vi "Init sm Measurement.vi"(4 "Enable Buffering (Enable)":bool, 5 "Sample Rate (1000 Hz)":i32=1000, 6 "Number of Acquisitions (100)":i32=100, 7 "Trigger Type (0:Untriggered)":u16(ring)=2 items=["Untriggered", "Software Triggered", "Hardware Triggered"], 8 "error in (no error)":errorcluster, 9 "Trigger Stop Condition (1:Edge Triggering)":u16(ring)=1 items=["Number of Acquisitions", "Edge Triggering"], 10 "Enable Unbuffered Data (Enabled)":bool=TRUE, 11 "Micron sm Digitizer in":refnum<class "Micron sm Digitizer.lvclass">) -> (0 "error out":errorcluster, 2 "Number of Sensors":u16[](array[numeric]), 3 "Micron sm Digitizer out":refnum<class "Micron sm Digitizer.lvclass">)   [LabVIEW 2024, in "Micron sm Digitizer.lvclass"]
uses:
  Micron sm Digitizer.lvclass
  D:/GitHub/NHMFL_Core/Libraries/Instruments/VISA Instrument/VISA Instrument.lvclass
  D:/GitHub/NHMFL_Core/Libraries/Instruments/Micron Optics/Micron Optics Driver/Micron Optics Driver.lvclass
  VISA Instrument/VISA Instrument.lvclass/VISA Instrument.ctl
  VISA Instrument/Read VISA resource.vi
  VISA Instrument/Write VISA resource.vi
  Micron sm Digitizer.lvclass/Micron sm Digitizer.ctl
  Micron Optics sm130/Micron Optics sm130.lvlib
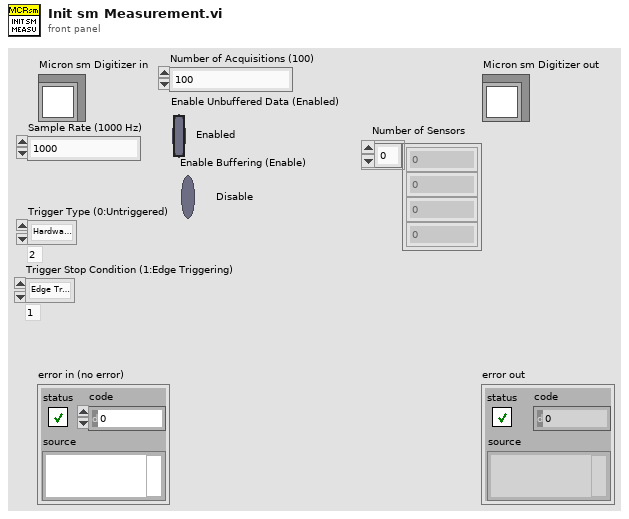
[diagram p1: front panel]
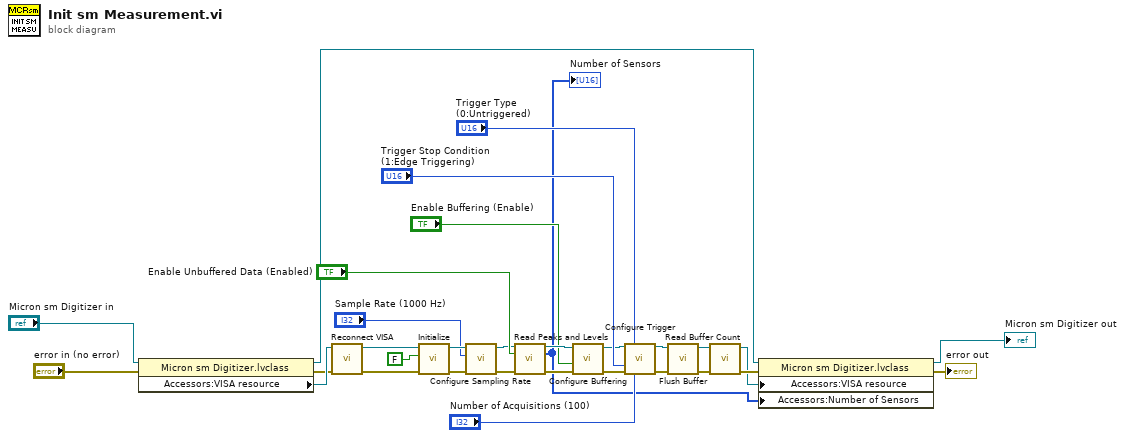
[diagram p0: block diagram]
diagram:
  n1 = property class="Micron sm Digitizer.lvclass"(reference="Micron sm Digitizer in", error in="error in (no error)") -> (reference out=w26:refnum<class "Micron sm Digitizer.lvclass">, error out=w2:errorcluster, "Accessors:VISA resource"=w4:refnum<visa-resource-name>)
  n2 = call "Reconnect VISA.vi"("error in"=w2, "VISA resource name"=w4) -> ("error out"=w1:errorcluster, "VISA resource name 2"=w3:refnum<visa-resource-name>)  [unwired: 8 in]
  n3 = call "Initialize.vi"("error in (no error)"=w1, "ID Query (True)"=FALSE, "VISA resource name"=w3) -> ("error out"=w9:errorcluster, "VISA resource name out"=w8:refnum<visa-resource-name>)  [unwired: 7 in]
  n4 = call "Configure Sampling Rate.vi"("error in (no error)"=w9, "Sample Rate (1000 Hz)"="Sample Rate (1000 Hz)", "VISA resource name"=w8) -> ("error out"=w7:errorcluster, "VISA resource name out"=w6:refnum<visa-resource-name>)  [unwired: 7 in]
  n5 = call "Read Peaks and Levels.vi"("VISA resource name"=w6, "Enable Unbuffered Data (Enabled)"="Enable Unbuffered Data (Enabled)", "error in (no error)"=w7) -> ("VISA resource name out"=w17:refnum<visa-resource-name>, "Number of Sensors"=w10:u16[], "error out"=w16:errorcluster)  [unwired: 4 in, 6 out]
  "Number of Sensors" <- w10
  n6 = call "Configure Buffering.vi"("error in (no error)"=w16, "Enable Buffering (Enable)"="Enable Buffering (Enable)", "VISA resource name"=w17) -> ("error out"=w22:errorcluster, "VISA resource name out"=w23:refnum<visa-resource-name>)  [unwired: 6 in, 1 out]
  n7 = call "Configure Trigger.vi"("VISA resource name"=w23, "Trigger Type (0:Untriggered)"="Trigger Type (0:Untriggered)", "Trigger Stop Condition (1:Edge Triggering)"="Trigger Stop Condition (1:Edge Triggering)", "error in (no error)"=w22, "Number of Acquisitions (100)"="Number of Acquisitions (100)") -> ("VISA resource name out"=w19:refnum<visa-resource-name>, "error out"=w18:errorcluster)  [unwired: 8 in, 1 out]
  n8 = call "Flush Buffer.vi"("error in (no error)"=w18, "VISA resource name"=w19) -> ("error out"=w24:errorcluster, "VISA resource name out"=w25:refnum<visa-resource-name>)  [unwired: 8 in]
  n9 = call "Read Buffer Count.vi"("error in"=w24, "VISA resource name"=w25) -> ("error out"=w21:errorcluster, "VISA resource name out"=w20:refnum<visa-resource-name>)  [unwired: 6 in, 2 out]
  n10 = property class="Micron sm Digitizer.lvclass"(reference=w26, error in=w21, "Accessors:VISA resource"=w20, "Accessors:Number of Sensors"=w10) -> (reference out=→"Micron sm Digitizer out":refnum<class "Micron sm Digitizer.lvclass">, error out=→"error out":errorcluster)
